vi "Logical String Array Sort.vi"(2 "Unsorted List":string[](array[string])) -> (16 "Sorted List":string[](array[string]))   [LabVIEW 2011, in "i3-oauth-logicalstringarraysort.lvlib"]
doc: "Sorts string arrays the way people normally would expect it to be sorted (treats numbers in the string as numbers, \"a9\" preceeds \"a12\" e.g.).\n\nBy Mads Toppe - 2005"
uses:
  i3-oauth-logicalstringarraysort.lvlib
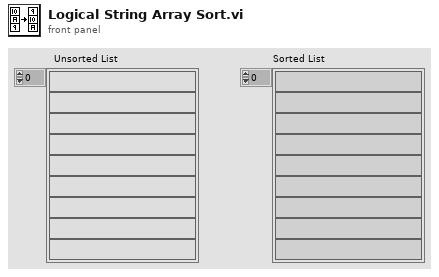
[diagram p1: front panel]
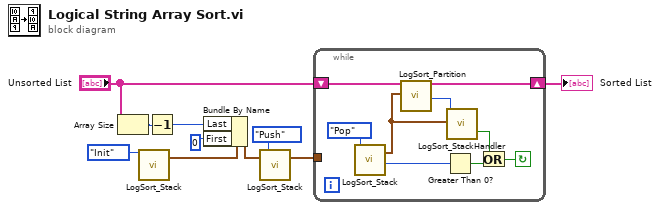
[diagram p0: block diagram]
diagram:
  n1 = Array Size(array="Unsorted List") -> (size(s)=w9:i32)
  n2 = call "LogSort_Stack.vi"("Function"=enum16{"Init", "Push", "Pop", "Size"}."Init") -> ("Indices"=w6:cluster{"First":i32, "Last":i32})  [unwired: 17 in, 1 out]
  n3 = Decrement(x=w9) -> (x-1=w8:i32)
  n4 = Bundle By Name(cluster=w6, "Last"=w8, "First"=0) -> (w5:cluster{"First":i32, "Last":i32})
  n5 = call "LogSort_Stack.vi"("Function"=enum16{"Init", "Push", "Pop", "Size"}."Push", "Indices"=w5) -> ("Indices"=w4:cluster{"First":i32, "Last":i32})  [unwired: 16 in, 1 out]
  n6 = while {
    tunnel: w4 -> [_]
    shift-left: "Unsorted List" -> [w19]
    shift-right: [w18] -> w3
    stop <- w13 continue-if-true
    n7 = call "LogSort_Stack.vi"("Function"=enum16{"Init", "Push", "Pop", "Size"}."Pop") -> ("Indices"=w11:cluster{"First":i32, "Last":i32}, "Size"=w15:i32)  [unwired: 17 in]
    n8 = call "LogSort_Partition.vi"("Array In"=w19, "Indices"=w11) -> ("Array Out"=w18:string[], "Split"=w17:i32)  [unwired: 16 in]
    n9 = Greater Than 0?(x=w15) -> (x > 0?=w14:bool)
    n10 = call "LogSort_StackHandler.vi"("Indices"=w11, "split"=w17) -> ("Stacked?"=w16:bool)  [unwired: 17 in]
    n11 = Or(x=w16, y=w14) -> (x .or. y?=w13:bool)
  }
  "Sorted List" <- w3
